vi "Joystick Circle Deadband (SubVI).vi"(9 "Joystick 1 Y Strafe":dbl, 10 "Joystick 1 X Forward/Back":dbl, 11 "Joystick Circular Deadband":dbl) -> (0 "In Deadband":bool, 2 "Joystick 1 Y Strafe":dbl, 3 "Joystick 1 X Forward/Back":dbl, 4 "joystickYInDeadband":bool, 6 "joystickXInDeadband":bool)   [LabVIEW 2020]
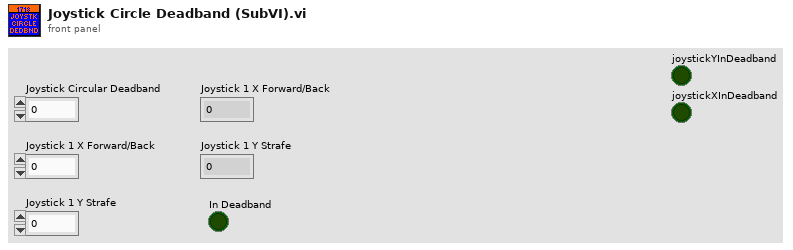
[diagram p1: front panel]
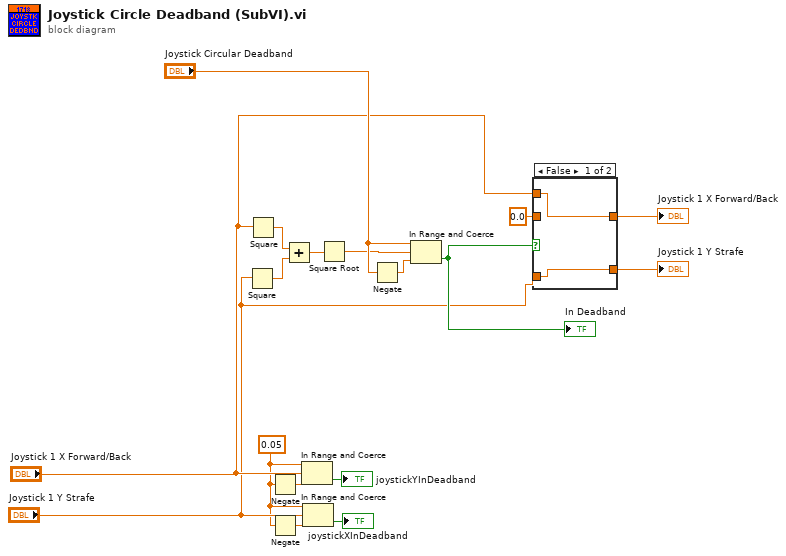
[diagram p0: block diagram]
diagram:
  w3 = 0.05 ("upper limit")
  n1 = Square(x="Joystick 1 Y Strafe") -> (x^2=w9:dbl)
  n2 = Square(x="Joystick 1 X Forward/Back") -> (x^2=w8:dbl)
  n3 = Negate(x=w3) -> (-x=w5:dbl)
  n4 = Negate(x=w3) -> (-x=w4:dbl)
  n5 = Add(x=w8, y=w9) -> (x+y=w10:dbl)
  n6 = In Range and Coerce(upper limit=w3, x="Joystick 1 X Forward/Back", lower limit=w5) -> (In Range?=→"joystickYInDeadband":bool)  [unwired: 1 out]
  n7 = In Range and Coerce(upper limit=w3, x="Joystick 1 Y Strafe", lower limit=w4) -> (In Range?=→"joystickXInDeadband":bool)  [unwired: 1 out]
  n8 = Square Root(x=w10) -> (sqrt(x)=w11:dbl)
  n9 = Negate(x="Joystick Circular Deadband") -> (-x=w12:dbl)
  n10 = In Range and Coerce(upper limit="Joystick Circular Deadband", x=w11, lower limit=w12) -> (In Range?=w14:bool)  [unwired: 1 out]
  "In Deadband" <- w14
  n11 = case shown="False" w14 {
    tunnel: 0.0 ("t") -> [_ w20]
    tunnel: [w18 w20] -> w17
    tunnel: [w19 w20] -> w16
    tunnel: "Joystick 1 X Forward/Back" -> [w18 _]
    tunnel: "Joystick 1 Y Strafe" -> [w19 _]
    frame False {
    }
    frame True {
    }
  }
  "Joystick 1 X Forward/Back" <- w17
  "Joystick 1 Y Strafe" <- w16
